vi "Write Config Params.vi"(8 "error in":errorcluster, 10 "Default Parameters":T1={"Common"={"Iteration Interval (s)"=0.001, "T0 (ns)"=0, "Priority"=100, "Processor"=-2, "Wait in Ready State"=TRUE}, "Amount of Channels"=0, "Address"=""} {"Common"."Iteration Interval (s)" format="%#_13g"}, 11 "Node in":refnum<class "AMS Climate Chamber Template.lvclass">) -> (0 "error out":errorcluster, 3 "Node out":refnum<class "AMS Climate Chamber Template.lvclass">)   [LabVIEW 2023, in "AMS Climate Chamber Template.lvlib" / "AMS Climate Chamber Template.lvclass"]
uses:
  AMS Climate Chamber Template.lvclass
  C:/Program Files/National Instruments/LabVIEW 2024/vi.lib/ADAS Replay HIL/Template Node/Plugin/Template Node/Template Node.lvclass
  Configuration Params.ctl
  <vilib>/ADAS Replay HIL/Template Node/Plugin/Template Node/Common Configuration Params.ctl
  AMS Climate Chamber Template.lvclass/AMS Climate Chamber Template.ctl
  <vilib>/ADAS Replay HIL/Template Node/Plugin/Template Node/Template Node.lvclass
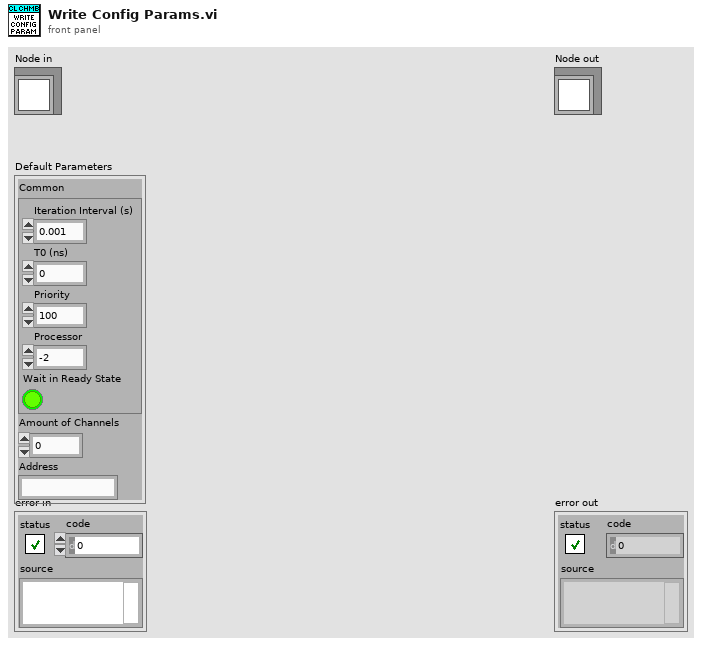
[diagram p1: front panel]
types:
  T1 = typedef "AMS Climate Chamber Template.lvlib/AMS Climate Chamber Template.lvclass/Configuration Params.ctl" = cluster{"Common":T2, "Amount of Channels":u32, "Address":string}
  T2 = typedef "Template Node.lvlib/Template Node.lvclass/Common Configuration Params.ctl" = cluster{"Iteration Interval (s)":dbl, "T0 (ns)":u64, "Priority":i32, "Processor":i32, "Wait in Ready State":bool}
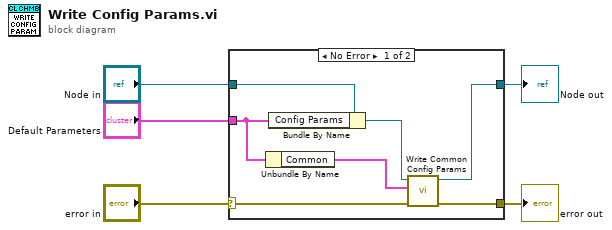
[diagram p0: block diagram]
diagram:
  n1 = case shown="No Error" "error in" {
    selector: "error in" -> [w12 w13]
    tunnel: [w10 w13] -> w4
    tunnel: [w8 w14] -> w2
    tunnel: "Node in" -> [w11 w14]
    tunnel: "Default Parameters" -> [w7 _]
    frame No Error {
      n2 = Unbundle By Name(w7) -> ("Common"=w6:T2)
      n3 = Bundle By Name(cluster=w11, "Config Params"=w7) -> (w9:refnum<class "AMS Climate Chamber Template.lvclass">)
      n4 = call <vilib>:"Write Common Config Params.vi"("error in"=w12, "Default Parameters"=w6, "Node in"=w9) -> ("error out"=w10:errorcluster, "Node out"=w8:refnum<class "AMS Climate Chamber Template.lvclass">)  [unwired: 7 in]
    }
    frame Error {
    }
  }
  "error out" <- w4
  "Node out" <- w2
